vi "Findallcolorsfornumbering_171213.vi"(9 "Size":i32, 10 "Input2Darray(SegmentedCircle)":u32[][](array[numeric]), 11 "Colors":u32[](array[numeric])) -> (3 "Numbering coordinates":cluster{i32, i32}[](array[cluster]))   [LabVIEW 2016]
panel:
  out "Help":picture
  out "Help 2":picture
  out "size 2":i32
  out "size count":i32
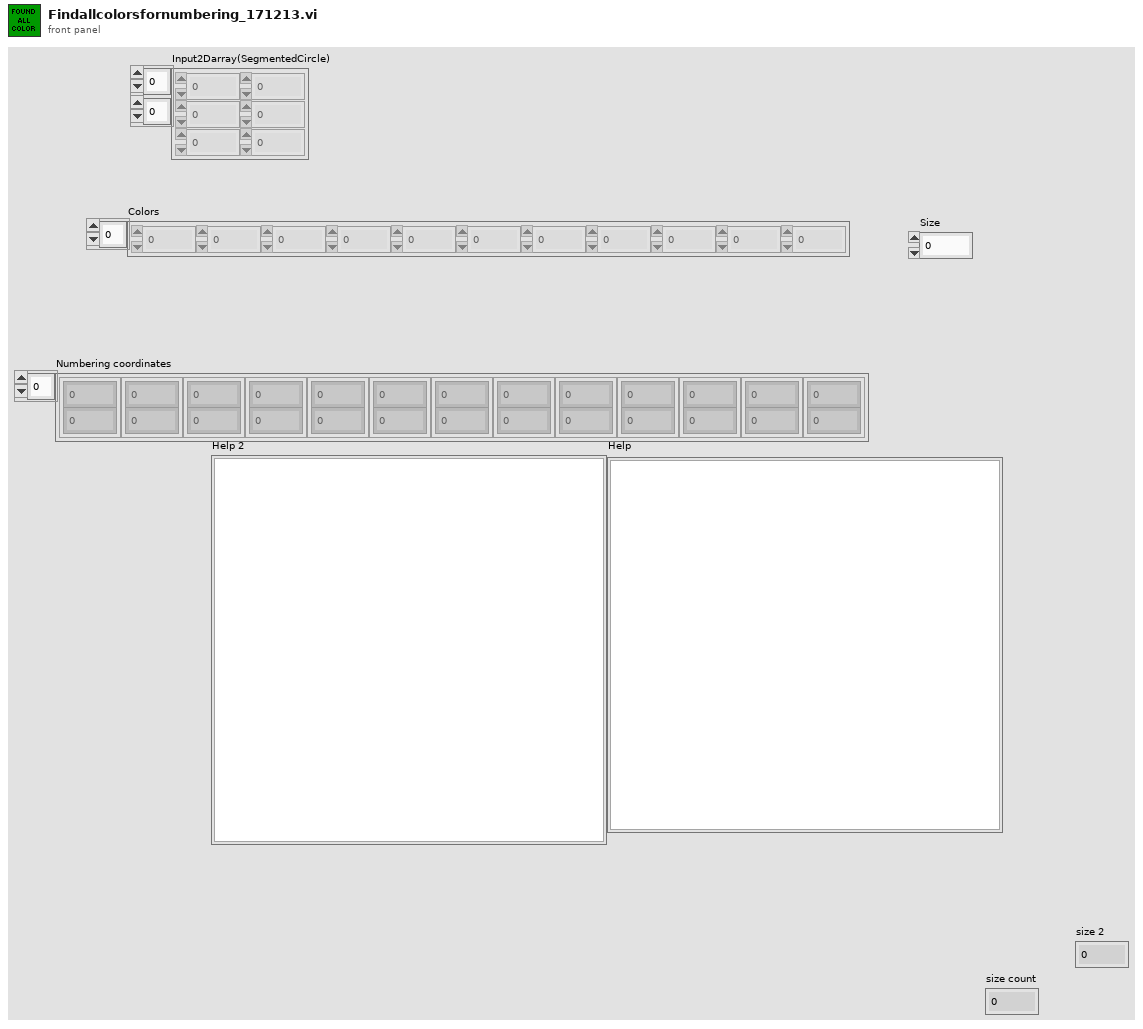
[diagram p1: front panel]
types:
  T1 = typedef "imagedata.ctl" = cluster{"image type":i32, "image depth":i32, "image":u8[], "mask":u8[], "colors":u32[], "Rectangle":cluster{"left":i16, "top":i16, "right":i16, "bottom":i16}}
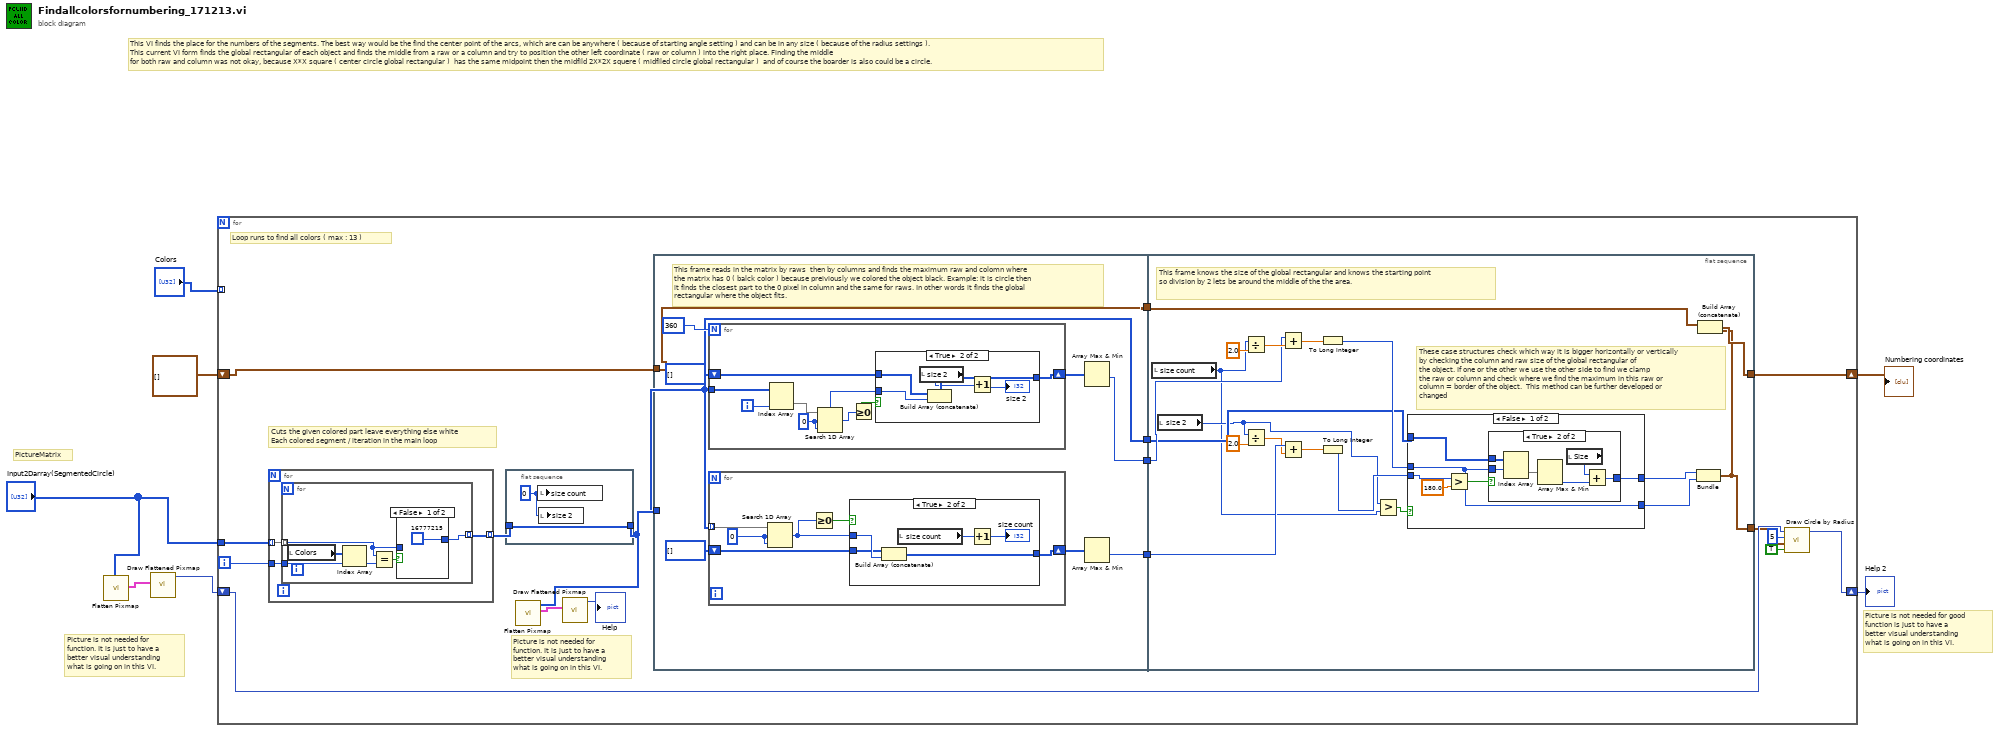
[diagram p0: block diagram]
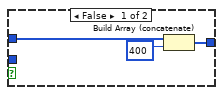
[diagram p2: hidden frame]
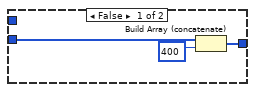
[diagram p3: hidden frame]
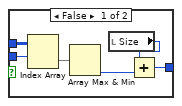
[diagram p4: hidden frame]
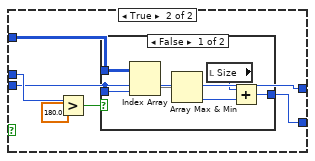
[diagram p5: hidden frame]
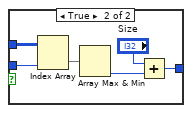
[diagram p6: hidden frame]
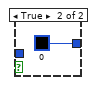
[diagram p7: hidden frame]
diagram:
  # "Picture is not needed for good\nfunction is just to have a \nbetter visual understanding \nwhat is going on in this VI."
  # "Picture is not needed for \nfunction. It is just to have a \nbetter visual understanding \nwhat is going on in this VI."
  # "PictureMatrix"
  # "This VI finds the place for the numbers of the segments. The best way would be the find the center point of the arcs, which are can be anywhere ( because of starting angle setting ) and can be in any size ( because of the radius settings ). \nThis current VI form finds the global rectangular of each object and finds the middle from a raw or a column and try to position the other left coordinate ( raw or column ) into the right place. Finding the middle \nfor both raw and column was not okay, because X*X square ( center circle global rectangular )  has the same midpoint then the midfild 2X*2X squere ( midfiled circle global rectangular )  and of course the boarder is also could be a circle."
  n1 = call <vilib>:"Flatten Pixmap.vi"("24-bit pixmap"="Input2Darray(SegmentedCircle)") -> ("image data"=w3:T1)  [unwired: 10 in]
  n2 = call <vilib>:"Draw Flattened Pixmap.vi"("image data"=w3) -> ("new picture"=w2:picture)  [unwired: 8 in]
  n3 = for {
    tunnel: "Input2Darray(SegmentedCircle)" -> [w21]
    tunnel: "Colors" -> [_] mode=indexing
    shift-right: [w18] -> w7
    shift-left: cluster{i32, i32}[] [] -> [w16]
    shift-right: [w15] -> w1
    shift-left: w2 -> [w14]
    i -> [w19]
    # "Loop runs to find all colors ( max : 13 )"
    # "Picture is not needed for \nfunction. It is just to have a \nbetter visual understanding \nwhat is going on in this VI."
    # "Cuts the given colored part leave everything else white\nEach colored segment / iteration in the main loop"
    n4 = for {
      tunnel: [w123] -> w20 mode=indexing
      tunnel: w21 -> [w122] mode=indexing
      tunnel: w19 -> [w121]
      n5 = for {
        tunnel: [w129] -> w123 mode=indexing
        tunnel: w122 -> [w128] mode=indexing
        tunnel: w121 -> [w124]
        n6 = local read "Colors"() -> (w126:u32[])
        n7 = Index Array(array=w126, index=w124) -> (element=w125:u32)
        n8 = Equal?(x=w128, y=w125) -> (x = y?=w127:bool)
        n9 = case shown="False" w127 {
          tunnel: [u32 16777215 u32 0 ("color(black)")] -> w129
          tunnel: w128 -> [_ _]
          frame False {
          }
          frame True {
          }
        }
      }
    }
    n10 = flat-sequence {
      tunnel: w20 -> [w26]
      tunnel: [w26] -> w10
      frame #0 {
        w25 = 0 ("size count")
        n11 = local write "size count"(w25) -> ()
        n12 = local write "size 2"(w25) -> ()
      }
    }
    n13 = call <vilib>:"Flatten Pixmap.vi"("24-bit pixmap"=w10) -> ("image data"=w9:T1)  [unwired: 10 in]
    n14 = call <vilib>:"Draw Flattened Pixmap.vi"("image data"=w9) -> ("new picture"=→"Help":picture)  [unwired: 8 in]
    n15 = flat-sequence {
      tunnel: w10 -> [w29]
      tunnel: [w34] -> w24
      tunnel: [w32] -> w23
      tunnel: [w29] -> w22
      tunnel: [w27] -> w17
      tunnel: w16 -> [w27]
      tunnel: w24 -> [w84]
      tunnel: w23 -> [w78]
      tunnel: w22 -> [w74]
      tunnel: [w71] -> w18
      tunnel: w17 -> [w70]
      tunnel: [w67] -> w13
      frame #0 {
        # "This frame reads in the matrix by raws  then by columns and finds the maximum raw and colomn where \nthe matrix has 0 ( balck color ) because preiviously we colored the object black. Example: it is circle then\nit finds the closest part to the 0 pixel in column and the same for raws. In other words it finds the global\nrectangular where the object fits."
        n16 = for {
          N: 360 -> [_]
          shift-right: [w41] -> w33
          shift-left: i32[] [] -> [w40]
          tunnel: w29 -> [w38]
          i -> [w36]
          w43 = 0 ("start index (0)")
          n17 = Index Array(array=w38, index (col)=w36) -> (element=w37:u32[])  [unwired: 1 in]
          n18 = Search 1D Array(1D array=w37, element=w43, start index (0)=w43) -> (index of element=w42:i32)
          n19 = Greater Or Equal To 0?(x=w42) -> (x >= 0?=w39:bool)
          n20 = case shown="True" w39 {
            tunnel: w42 -> [_ w50]
            tunnel: [w45 w51] -> w41
            tunnel: w40 -> [w46 w49]
            frame False {
              n21 = Build Array (concatenate)(w46, 400 ("start index (0)")) -> (w45:i32[])
            }
            frame True {
              n22 = local read "size 2"() -> (w48:i32)
              n23 = Build Array (concatenate)(w49, w50) -> (w51:i32[])
              n24 = Increment(x=w48) -> (x+1=→"size 2":i32)
            }
          }
        }
        n25 = for {
          tunnel: w29 -> [w52] mode=indexing
          shift-right: [w55] -> w28
          shift-left: i32[] [] -> [w54]
          w57 = 0 ("start index (0)")
          n26 = Search 1D Array(1D array=w52, element=w57, start index (0)=w57) -> (index of element=w56:i32)
          n27 = Greater Or Equal To 0?(x=w56) -> (x >= 0?=w53:bool)
          n28 = case shown="True" w53 {
            tunnel: w56 -> [_ w64]
            tunnel: [w59 w65] -> w55
            tunnel: w54 -> [w60 w63]
            frame False {
              n29 = Build Array (concatenate)(w60, 400 ("start index (0)")) -> (w59:i32[])
            }
            frame True {
              n30 = Build Array (concatenate)(w63, w64) -> (w65:i32[])
              n31 = local read "size count"() -> (w62:i32)
              n32 = Increment(x=w62) -> (x+1=→"size count":i32)
            }
          }
        }
        n33 = Array Max & Min(array=w33) -> (min value=w32:i32)  [unwired: 3 out]
        n34 = Array Max & Min(array=w28) -> (min value=w34:i32)  [unwired: 3 out]
      }
      frame #1 {
        # "These case structures check which way it is bigger horizontally or vertically \nby checking the column and raw size of the global rectangular of \nthe object. If one or the other we use the other side to find we clamp\nthe raw or column and check where we find the maximum in this raw or \ncolumn = border of the object.  This method can be further developed or \nchanged"
        # "This frame knows the size of the global rectangular and knows the starting point \nso division by 2 lets be around the middle of the the area."
        n35 = local read "size count"() -> (w68:i32)
        n36 = local read "size 2"() -> (w69:i32)
        n37 = Divide(x=w68, y=2.0) -> (x/y=w80:dbl)
        n38 = Divide(x=w69, y=2.0) -> (x/y=w82:dbl)
        n39 = Add(x=w78, y=w80) -> (x+y=w76:dbl)
        n40 = Add(x=w84, y=w82) -> (x+y=w81:dbl)
        n41 = To Long Integer(number=w76) -> (32bit integer=w75:i32)
        n42 = To Long Integer(number=w81) -> (32bit integer=w77:i32)
        n43 = Greater?(x=w69, y=w68) -> (0:w66:bool)
        n44 = case shown="False" w66 {
          tunnel: w77 -> [w87 w103]
          tunnel: [w90 w103] -> w73
          tunnel: w75 -> [w85 w105]
          tunnel: [w85 w108] -> w72
          tunnel: w74 -> [w86 w104]
          frame False {
            n45 = Greater?(x=w87, y=180.0) -> (0:w88:bool)
            n46 = case shown="True" w88 {
              tunnel: [w92 w98] -> w90
              tunnel: w86 -> [w95 w102]
              tunnel: w85 -> [w96 w101]
              frame False {
                n47 = Index Array(array=w95, index (row)=w96) -> (element=w94:u32[])  [unwired: 1 in]
                n48 = Array Max & Min(array=w94) -> (min index (indices)=w93:i32)  [unwired: 3 out]
                n49 = local read "Size"() -> (w91:i32)
                n50 = Add(x=w91, y=w93) -> (x+y=w92:i32)
              }
              frame True {
                n51 = Index Array(array=w102, index (row)=w101) -> (element=w100:u32[])  [unwired: 1 in]
                n52 = Array Max & Min(array=w100) -> (min index (indices)=w99:i32)  [unwired: 3 out]
                n53 = local read "Size"() -> (w97:i32)
                n54 = Add(x=w97, y=w99) -> (x+y=w98:i32)
              }
            }
          }
          frame True {
            n55 = Greater?(x=w105, y=180.0) -> (0:w107:bool)
            n56 = case shown="False" w107 {
              tunnel: [w110 w116] -> w108
              tunnel: w104 -> [w114 w120]
              tunnel: w103 -> [w113 w118]
              frame False {
                n57 = Index Array(array=w114, index (col)=w113) -> (element=w111:u32[])  [unwired: 1 in]
                n58 = Array Max & Min(array=w111) -> (min index (indices)=w112:i32)  [unwired: 3 out]
                n59 = local read "Size"() -> (w109:i32)
                n60 = Add(x=w109, y=w112) -> (x+y=w110:i32)
              }
              frame True {
                n61 = Index Array(array=w120, index (col)=w118) -> (element=w119:u32[])  [unwired: 1 in]
                n62 = Array Max & Min(array=w119) -> (min index (indices)=w117:i32)  [unwired: 3 out]
                n63 = Add(x="Size", y=w117) -> (x+y=w116:i32)
              }
            }
          }
        }
        n64 = Bundle(w73, w72) -> (w67:cluster{i32, i32})  [unwired: 1 in]
        n65 = Build Array (concatenate)(w70, w67) -> (w71:cluster{i32, i32}[])
      }
    }
    n66 = call <vilib>:"Draw Circle by Radius.vi"("fill?(F)"=TRUE, "pixel center"=w13, "radius"=i16 5, "picture"=w14) -> ("new picture"=w15:picture)  [unwired: 7 in]
  }
  "Numbering coordinates" <- w7
  "Help 2" <- w1
